vi "testSameError.vi"() -> ()   [LabVIEW 2019, in "AssertionTest.lvlib" / "AssertErrorCode.lvlib"]
uses:
  AssertErrorCode.lvlib
  c2093d00-4b88-487e-b182-b5504d5fada5.vi
  <vilib>/Utility/error.llb/Error Cluster From Error Code.vi
  Constraint/IsEqual/Create.vi
  <vilib>/ErrorRing/Error Ring.xnode
  Constraint/IsEqual/IsEqual.lvclass
  Assertion/Assertion.lvlib
panel:
  out "error out":errorcluster
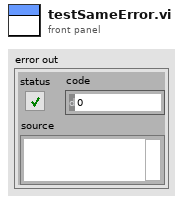
[diagram p1: front panel]
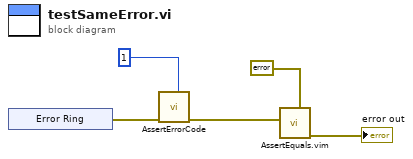
[diagram p0: block diagram]
diagram:
  n1 = xnode "Error Ring"() -> ("error out"=w4:errorcluster)
  n2 = call "AssertErrorCode.vi"("Expected"=1, "error in (no error)"=w4) -> ("error out"=w2:errorcluster)  [unwired: 9 in]
  n3 = call "AssertEquals.vim"("Expected"=errorcluster {"status"=FALSE, "code"=0, "source"=""} ("error constant"), "Actual"=w2) -> ("error out"=→"error out":errorcluster)  [unwired: 9 in]
